vi "Save Data (SubVI)_lxy.vi"(10 "path":path, 11 "队列输入":refnum<queue>) -> ()   [LabVIEW 2019]
uses:
  <vilib>/Utility/file.llb/Write Delimited Spreadsheet (string).vi
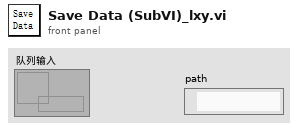
[diagram p1: front panel]
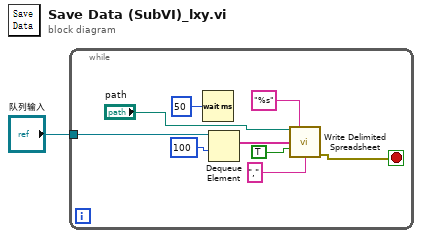
[diagram p0: block diagram]
diagram:
  n1 = while {
    tunnel: "队列输入" -> [w10]
    stop <- w9 stop-if-true
    n2 = Wait (ms)(milliseconds to wait=u32 50 ("等待时间（毫秒）")) -> ()  [unwired: 1 out]
    n3 = Dequeue Element(queue=w10, timeout in ms (-1)=100 ("超时毫秒(-1)")) -> (element=w3:string[])  [unwired: 1 in, 3 out]
    n4 = call-poly <vilib>:"Write Delimited Spreadsheet.vi"("file path (dialog if empty)"="path", "format (%s)"="%s" ("format (%.3f)"), "1D data"=w3, "append to file? (new file:F)"=TRUE, "delimiter (\\t)"="," ("delimiter (\\t)")) -> ("error out"=w9:errorcluster)  [unwired: 9 in, 1 out]
  }
